vi "Image Processing Main Timing.vi"() -> ()   [LabVIEW 2009]
uses:
  <vilib>/vision/driver/NI_Vision_Acquisition_Software.lvlib
  <vilib>/vision/driver/IMAQdx.llb/IMAQdx Acquisition Mode.ctl
  <vilib>/userDefined/High Color/IMAQdx.ctl
panel:
  out "Total time":u32
  out "Create SICK":u32
  out "Compare to masks":u32
  out "Extract lines":u32
  out "Image Aquisition":u32
  out "Sick array":i32[](array[numeric])
  in  "stop":bool
  out "Right Camera Input":T1(plugin-control)
  out "Left Camera Input":T1(plugin-control)
  out "Right Camera Output":T1(plugin-control)
  out "Left Camera Output":T1(plugin-control)
  in  "IMAQdx Session Right":T2="cam1" caption="Session In"
  in  "IMAQdx Session Left":T2="cam0" caption="Session In"
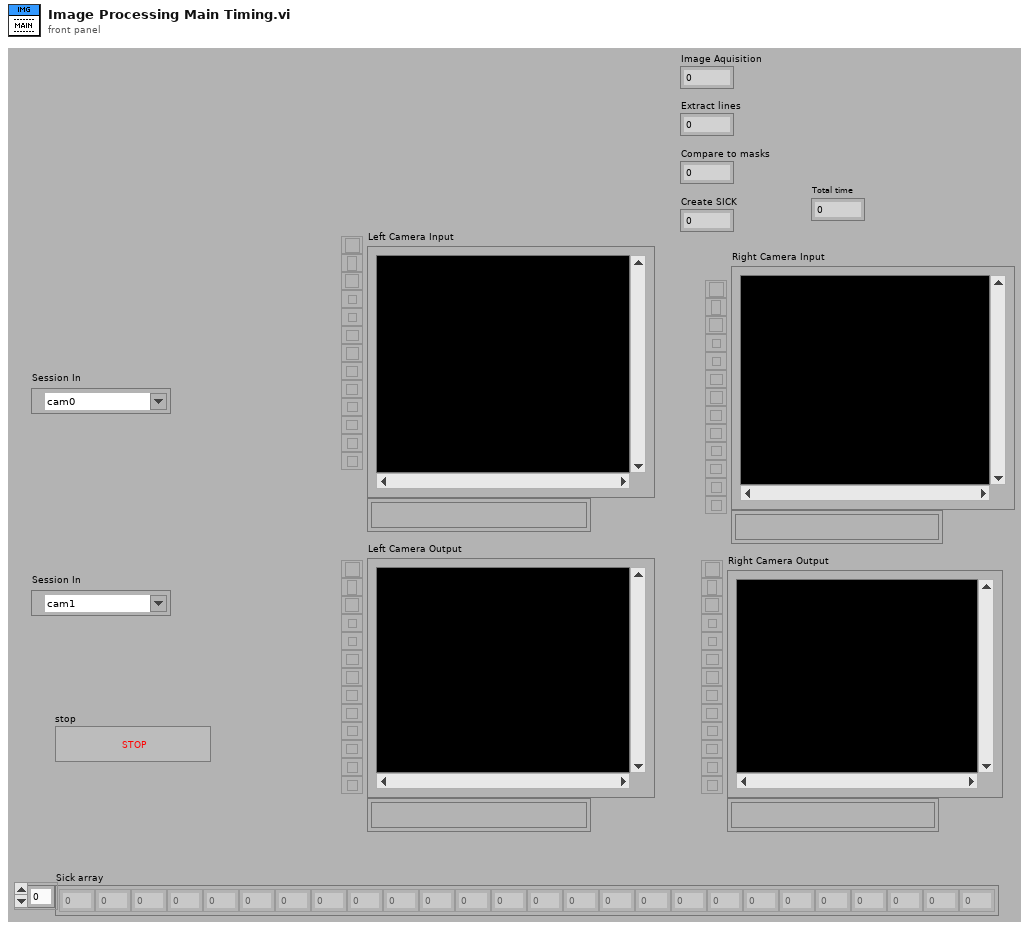
[diagram p1: front panel]
types:
  T1 = typedef "IMAQ Image.ctl" = refnum<image>
  T2 = typedef "IMAQdx.ctl" = refnum<k21>
  T3 = typedef "NI_Vision_Acquisition_Software.lvlib/IMAQdx Acquisition Mode.ctl" = enum32{"One Shot", "Continuous"}
  T4 = typedef "Image Type" = u32
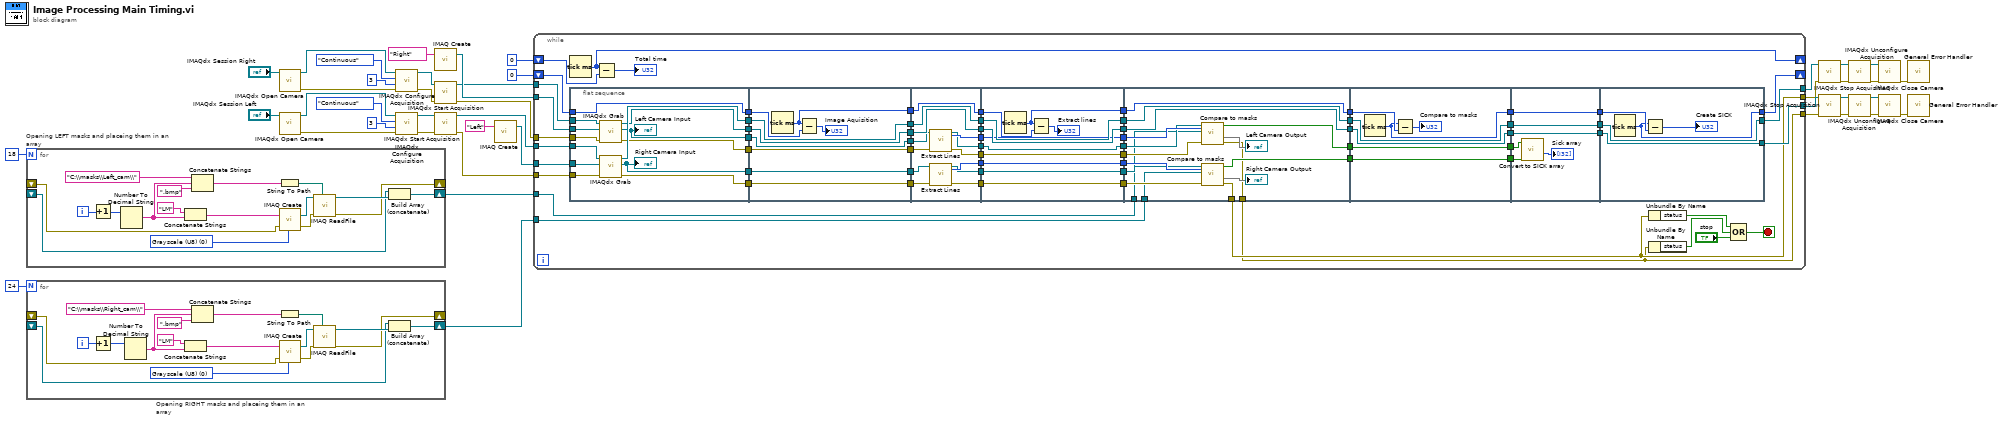
[diagram p0: block diagram]
diagram:
  n1 = for "Opening LEFT masks and placeing them in an array" {
    N: 18 -> [_]
    shift-right: [w53] -> w5
    shift-left: _ -> [w52]
    shift-right: [w51] -> _
    shift-left: _ -> [w50]
    i -> [w57]
    w55 = T4 0 items=["Grayscale (U8)", "Grayscale (I16)", "Grayscale (SGL)", "Complex (CSG)", "RGB (U32)", "HSL (U32)", "RGB (U64)", "Grayscale (U16)"] ("Image Type")
    n2 = Increment(x=w57) -> (x+1=w56:i32)
    n3 = Number To Decimal String(number=w56) -> (decimal integer string=w47:string)  [unwired: 1 in]
    n4 = Concatenate Strings("LM" ("element"), w47) -> (w43:string)
    n5 = Concatenate Strings("C:\\masks\\Left_cam\\", w47, ".bmp") -> (w44:string)
    n6 = String To Path(string=w44) -> (path=w45:path)
    n7 = call "IMAQ Create"("Image Name"=w43, "Image Type"=w55, "error in (no error)"=w50) -> ("New Image"=w58:T1, "error out"=w59:errorcluster)  [unwired: 2 in]
    n8 = call "IMAQ ReadFile"("File Path"=w45, "error in (no error)"=w59, "Image"=w58) -> ("error out"=w51:errorcluster, "Image Out"=w54:T1)  [unwired: 4 in, 3 out]
    n9 = Build Array (concatenate)(w52, w54) -> (w53:T1[])
  }
  n10 = for "Opening RIGHT masks and placeing them in an array" {
    N: 24 -> [_]
    shift-right: [w70] -> w7
    shift-left: _ -> [w69]
    shift-right: [w68] -> _
    shift-left: _ -> [w67]
    i -> [w74]
    w72 = T4 0 items=["Grayscale (U8)", "Grayscale (I16)", "Grayscale (SGL)", "Complex (CSG)", "RGB (U32)", "HSL (U32)", "RGB (U64)", "Grayscale (U16)"] ("Image Type")
    n11 = Increment(x=w74) -> (x+1=w73:i32)
    n12 = Number To Decimal String(number=w73) -> (decimal integer string=w64:string)  [unwired: 1 in]
    n13 = Concatenate Strings("LM" ("element"), w64) -> (w60:string)
    n14 = Concatenate Strings("C:\\masks\\Right_cam\\", w64, ".bmp") -> (w61:string)
    n15 = String To Path(string=w61) -> (path=w62:path)
    n16 = call "IMAQ Create"("Image Name"=w60, "Image Type"=w72, "error in (no error)"=w67) -> ("New Image"=w75:T1, "error out"=w76:errorcluster)  [unwired: 2 in]
    n17 = call "IMAQ ReadFile"("File Path"=w62, "error in (no error)"=w76, "Image"=w75) -> ("error out"=w68:errorcluster, "Image Out"=w71:T1)  [unwired: 4 in, 3 out]
    n18 = Build Array (concatenate)(w69, w71) -> (w70:T1[])
  }
  n19 = call <vilib>:"IMAQdx Open Camera.vi"("Session In"="IMAQdx Session Right") -> ("error out"=w29:errorcluster, "Session Out"=w30:T2)  [unwired: 2 in, 7 out]
  n20 = call <vilib>:"IMAQdx Open Camera.vi"("Session In"="IMAQdx Session Left") -> ("error out"=w37:errorcluster, "Session Out"=w36:T2)  [unwired: 2 in, 7 out]
  n21 = call <vilib>:"IMAQdx Configure Acquisition.vi"("error in"=w29, "Number of Buffers"=u32 3, "Continuous?"=IMAQdx_Acquisition_Mode."Continuous", "Session In"=w30) -> ("error out"=w28:errorcluster, "Session Out"=w31:T2)  [unwired: 1 in, 5 out]
  n22 = call <vilib>:"IMAQdx Configure Acquisition.vi"("error in"=w37, "Number of Buffers"=u32 3, "Continuous?"=IMAQdx_Acquisition_Mode."Continuous", "Session In"=w36) -> ("error out"=w38:errorcluster, "Session Out"=w35:T2)  [unwired: 1 in, 5 out]
  n23 = call "IMAQ Create"("Image Name"="Right") -> ("New Image"=w41:T1)  [unwired: 4 in, 1 out]
  n24 = call <vilib>:"IMAQdx Start Acquisition.vi"("error in"=w28, "Session In"=w31) -> ("error out"=w26:errorcluster, "Session Out"=w27:T2)  [unwired: 8 out]
  n25 = call <vilib>:"IMAQdx Start Acquisition.vi"("error in"=w38, "Session In"=w35) -> ("error out"=w33:errorcluster, "Session Out"=w34:T2)  [unwired: 8 out]
  n26 = call "IMAQ Create"("Image Name"="Left") -> ("New Image"=w40:T1)  [unwired: 4 in, 1 out]
  n27 = while {
    tunnel: w34 -> [w142]
    tunnel: w40 -> [w141]
    tunnel: w26 -> [w140]
    tunnel: w27 -> [w139]
    tunnel: w33 -> [w138]
    tunnel: w41 -> [w137]
    tunnel: [w136] -> w13
    tunnel: [w135] -> w19
    tunnel: w7 -> [w134]
    tunnel: w5 -> [w133]
    tunnel: [w127] -> w3
    tunnel: [w128] -> w4
    shift-right: [w77] -> _
    shift-left: u32 0 -> [w132]
    shift-right: [w123] -> _
    shift-left: u32 0 ("millisecond timer value") -> [w124]
    stop <- w126 stop-if-true
    n28 = Tick Count (ms)() -> (millisecond timer value=w123:u32)
    n29 = flat-sequence {
      tunnel: w142 -> [w155]
      tunnel: w141 -> [w154]
      tunnel: w140 -> [w153]
      tunnel: w139 -> [w152]
      tunnel: w138 -> [w151]
      tunnel: w137 -> [w150]
      tunnel: [w149] -> w122
      tunnel: [w148] -> w120
      tunnel: [w147] -> w118
      tunnel: [w146] -> w116
      tunnel: [w145] -> w114
      tunnel: [w144] -> w112
      tunnel: w132 -> [w143]
      tunnel: [w143] -> w110
      tunnel: w122 -> [w164]
      tunnel: [w164] -> w121
      tunnel: w120 -> [w163]
      tunnel: [w163] -> w119
      tunnel: w118 -> [w162]
      tunnel: [w162] -> w117
      tunnel: w116 -> [w161]
      tunnel: [w161] -> w115
      tunnel: w114 -> [w160]
      tunnel: [w160] -> w113
      tunnel: w112 -> [w159]
      tunnel: [w159] -> w111
      tunnel: w110 -> [w157]
      tunnel: [w156] -> w92
      tunnel: w121 -> [w177]
      tunnel: w119 -> [w176]
      tunnel: w117 -> [w173]
      tunnel: w115 -> [w174]
      tunnel: w113 -> [w175]
      tunnel: w111 -> [w172]
      tunnel: [w177] -> w109
      tunnel: [w176] -> w107
      tunnel: [w171] -> w105
      tunnel: [w170] -> w103
      tunnel: [w169] -> w101
      tunnel: [w168] -> w99
      tunnel: [w167] -> w97
      tunnel: [w166] -> w95
      tunnel: [w165] -> w93
      tunnel: w92 -> [w165]
      tunnel: w109 -> [w188]
      tunnel: [w188] -> w108
      tunnel: w107 -> [w187]
      tunnel: [w187] -> w106
      tunnel: w105 -> [w186]
      tunnel: [w186] -> w104
      tunnel: w103 -> [w185]
      tunnel: [w185] -> w102
      tunnel: w101 -> [w184]
      tunnel: [w184] -> w100
      tunnel: w99 -> [w183]
      tunnel: [w183] -> w98
      tunnel: w97 -> [w182]
      tunnel: [w182] -> w96
      tunnel: w95 -> [w181]
      tunnel: [w181] -> w94
      tunnel: w93 -> [w179]
      tunnel: [w178] -> w82
      tunnel: w108 -> [w205]
      tunnel: w106 -> [w204]
      tunnel: w104 -> [w203]
      tunnel: w102 -> [w202]
      tunnel: w100 -> [w201]
      tunnel: w98 -> [w200]
      tunnel: w96 -> [w199]
      tunnel: w94 -> [w198]
      tunnel: w134 -> [w197]
      tunnel: w133 -> [w196]
      tunnel: [w205] -> w91
      tunnel: [w204] -> w89
      tunnel: [w195] -> w87
      tunnel: [w194] -> w85
      tunnel: [w191] -> w127
      tunnel: [w190] -> w128
      tunnel: [w189] -> w83
      tunnel: w82 -> [w189]
      tunnel: w91 -> [w212]
      tunnel: [w212] -> w90
      tunnel: w89 -> [w211]
      tunnel: [w211] -> w88
      tunnel: w87 -> [w210]
      tunnel: [w210] -> w86
      tunnel: w85 -> [w209]
      tunnel: [w209] -> w84
      tunnel: w83 -> [w207]
      tunnel: [w206] -> w78
      tunnel: w90 -> [w218]
      tunnel: w88 -> [w217]
      tunnel: w86 -> [w215]
      tunnel: w84 -> [w214]
      tunnel: [w218] -> w81
      tunnel: [w217] -> w80
      tunnel: [w213] -> w79
      tunnel: w78 -> [w213]
      tunnel: [w222] -> w135
      tunnel: [w223] -> w136
      tunnel: w81 -> [w223]
      tunnel: w80 -> [w222]
      tunnel: w79 -> [w220]
      tunnel: [w219] -> w77
      frame #0 {
        n30 = call <vilib>:"IMAQdx Grab.vi"("error in"=w153, "Image In"=w150, "Session In"=w152) -> ("error out"=w146:errorcluster, "Image Out"=w145:T1, "Session Out"=w148:T2)  [unwired: 5 in, 1 out]
        "Left Camera Input" <- w145
        n31 = call <vilib>:"IMAQdx Grab.vi"("error in"=w151, "Image In"=w154, "Session In"=w155) -> ("error out"=w147:errorcluster, "Image Out"=w144:T1, "Session Out"=w149:T2)  [unwired: 5 in, 1 out]
        "Right Camera Input" <- w144
      }
      frame #1 {
        n32 = Tick Count (ms)() -> (millisecond timer value=w156:u32)
        n33 = Subtract(x=w156, y=w157) -> (x-y=→"Image Aquisition":u32)
      }
      frame #2 {
        n34 = call "Extract Lines.vi"("error in (no error)"=w174, "Image Src"=w175) -> ("error out"=w169:errorcluster, "Image Out"=w168:T1, "Extraction mode"=w170:i32)  [unwired: 6 in, 1 out]
        n35 = call "Extract Lines.vi"("error in (no error)"=w173, "Image Src"=w172) -> ("error out"=w166:errorcluster, "Image Out"=w167:T1, "Extraction mode"=w171:i32)  [unwired: 6 in, 1 out]
      }
      frame #3 {
        n36 = Tick Count (ms)() -> (millisecond timer value=w178:u32)
        n37 = Subtract(x=w178, y=w179) -> (x-y=→"Extract lines":u32)
      }
      frame #4 {
        n38 = call "Compare to masks.vi"("Number of Particles1"=w202, "error in (no error)"=w201, "Mask array"=w196, "Image Src"=w200) -> ("Final error out"=w191:errorcluster, 1:→"Left Camera Output", "Marked Regions"=w194:bool[])  [unwired: 5 in]
        n39 = call "Compare to masks.vi"("Number of Particles1"=w203, "error in (no error)"=w198, "Mask array"=w197, "Image Src"=w199) -> ("Final error out"=w190:errorcluster, 1:→"Right Camera Output", "Marked Regions"=w195:bool[])  [unwired: 5 in]
      }
      frame #5 {
        n40 = Tick Count (ms)() -> (millisecond timer value=w206:u32)
        n41 = Subtract(x=w206, y=w207) -> (x-y=→"Compare to masks":u32)
      }
      frame #6 {
        n42 = call "Convert to SICK array.vi"("Left Regions"=w215, "Right Regions"=w214) -> ("Sick array"=→"Sick array":u16[])  [unwired: 9 in]
      }
      frame #7 {
        n43 = Tick Count (ms)() -> (millisecond timer value=w219:u32)
        n44 = Subtract(x=w219, y=w220) -> (x-y=→"Create SICK":u32)
      }
    }
    n45 = Subtract(x=w123, y=w124) -> (x-y=→"Total time":u32)
    n46 = Unbundle By Name(w128) -> ("status"=w130:bool)
    n47 = Unbundle By Name(w127) -> ("status"=w131:bool)
    n48 = Compound Arithmetic op=OR(w130, w131, "stop") -> (w126:bool)
  }
  n49 = call <vilib>:"IMAQdx Stop Acquisition.vi"("error in"=w4, "Session In"=w13) -> ("error out"=w16:errorcluster, "Session Out"=w17:T2)  [unwired: 8 out]
  n50 = call <vilib>:"IMAQdx Stop Acquisition.vi"("error in"=w3, "Session In"=w19) -> ("error out"=w22:errorcluster, "Session Out"=w21:T2)  [unwired: 8 out]
  n51 = call <vilib>:"IMAQdx Unconfigure Acquisition.vi"("error in"=w16, "Session In"=w17) -> ("error out"=w15:errorcluster, "Session Out"=w14:T2)  [unwired: 8 out]
  n52 = call <vilib>:"IMAQdx Unconfigure Acquisition.vi"("error in"=w22, "Session In"=w21) -> ("error out"=w23:errorcluster, "Session Out"=w24:T2)  [unwired: 8 out]
  n53 = call <vilib>:"IMAQdx Close Camera.vi"("error in"=w15, "Session In"=w14) -> ("error out"=w18:errorcluster)  [unwired: 9 out]
  n54 = call <vilib>:"IMAQdx Close Camera.vi"("error in"=w23, "Session In"=w24) -> ("error out"=w20:errorcluster)  [unwired: 9 out]
  n55 = call <vilib>:"General Error Handler.vi"("error in (no error)"=w18) -> ()  [unwired: 1 in, 14 out]
  n56 = call <vilib>:"General Error Handler.vi"("error in (no error)"=w20) -> ()  [unwired: 1 in, 14 out]
